vi "Transport Optimization Using Linear Programming.vi"() -> ()   [LabVIEW 2023]
doc: "Uses the Linear Programming Simplex Method VI to determine the number of units that company x transports to trader y."
panel:
  out "Error Status":bool
  in  "Tab Control":T1(tab)
  in  "Producers":cluster{"name":string, "produced units":dbl}[](array[cluster])=[{"name"="company A", "produced units"=213.0}, {"name"="company B", "produced units"=342.0}, {"name"="company C", "produced units"=543.0}, {"name"="company D", "produced units"=154.0}] {"produced units" format="%#.6g"}
  in  "Traders":cluster{"name":string, "needed units":dbl}[](array[cluster])=[{"name"="trader 1", "needed units"=564.0}, {"name"="trader 2", "needed units"=123.0}, {"name"="trader 3", "needed units"=234.0}, {"name"="trader 4", "needed units"=331.0}] {"needed units" format="%#.6g"}
  out "sum of produced units":dbl format="%#.6g"
  out "sum of needed units":dbl format="%#.6g"
  in  "Transport Costs (currency)":dbl[][](array[numeric])=[[213.0, 301.0, 453.0, 743.0], [99.0, 612.0, 209.0, 543.0], [123.0, 109.0, 453.0, 435.0], [129.0, 234.0, 432.0, 876.0]] min=0.0 format="%#.6g"
  out "Producers names":string[](array[string])
  out "Traders names":string[](array[string])
  out "minimal cost":dbl
  out "What delivers producer to trader #?":dbl[](graph)
  in  "Producer selector":u16(ring) items=["company A", "company B", "company C", "company D"]
  in  "Trader selector":u16(ring) items=["trader 1", "trader 2", "trader 3", "trader 4"]
  out "What gets trader from company #?":dbl[](graph)
  out "production":dbl
  out "delivery":dbl
  out "solution":dbl[][](array[numeric]) format="%#.2g"
  in  "Stop":bool
  # "Overview: Uses the Linear Programming Simplex Method VI to determine the number of units that company x transports to trader y with the firm M.\nRequirements: LabVIEW Full Development System\nInstructions: \n1. Specify the number of units in the Production and Consumption tab. Also, define the cost of transportation from each producer to each trader in the Transport Cost tab.\n2. Run the VI and verify the solution of this problem in the Solution tab. Use the Producer selector and Trader selector rings to analyze company and trader costs and minimum possible cost.\n3. Click Stop to stop the VI."
  # "Trader 1"
  # "Costs"
  # "P1->T1"
  # "Producer 1"
  # "P1->T2"
  # "Trader 2"
  # "Producer 2"
  # "P2->T1"
  # "P2->T2"
  # "Transporter"
  # "produced units"
  # "needed units"
  # "Constraint - every unit produced is consumed."
  # "The Transportation Problem is a linear programming problem where the lowest cost of transportation between Producer and Trader is obtained, taking into account the maximum throughput. The formulation is:\n\nMinimize: Sum ( c11.x11 + c12.x12 + .. + cmn.xmn).\nSubject to:\nx11 + x12 + ... + x1n <= b1;\n......\nxm1 + xm2 + ... + xmn <= bm;\nx11 + x12 + ... + xm1 >= a1;\n.......\nxm1 + xm2 + ... + xmn >= an;\nwhere:\nm: number of producers.\nn: number of traders."
  # "Traders"
  # "0"
  # "1"
  # "2"
  # "3"
  # "0"
  # "Producers"
  # "1"
  # "2"
  # "3"
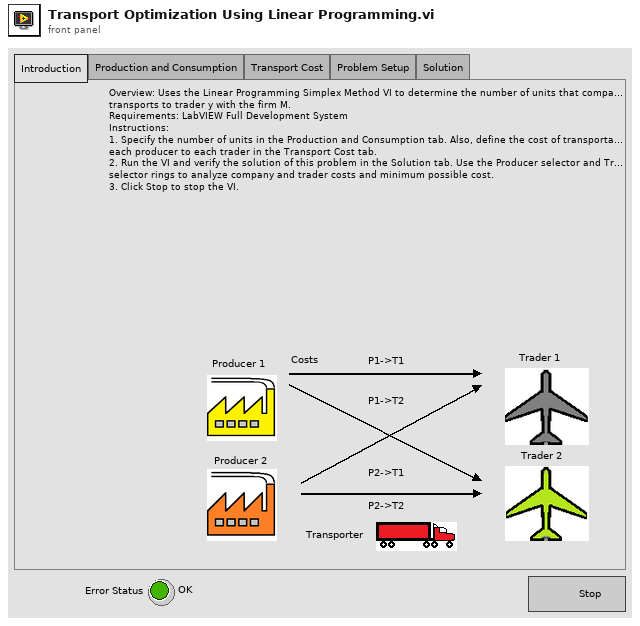
[diagram p1: front panel]
types:
  T1 = enum32{"Introduction", "Production and Consumption", "Transport Cost", "Problem Setup", "Solution"}
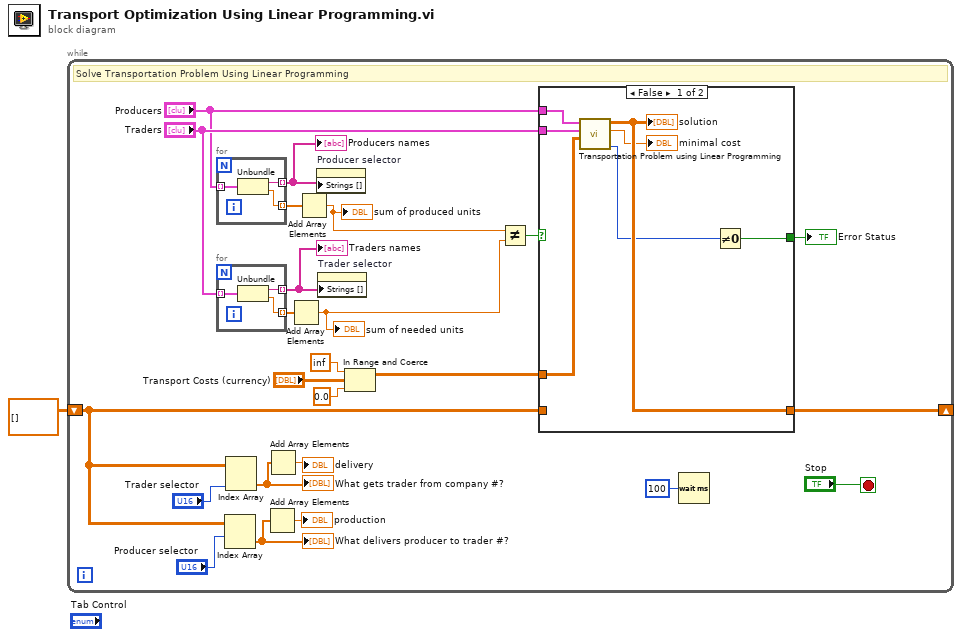
[diagram p0: block diagram]
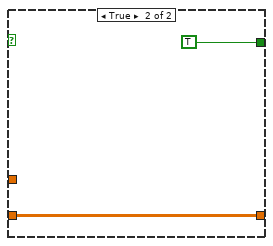
[diagram p2: hidden frame]
diagram:
  n1 = while {
    shift-left: dbl[][] [] ("Solution") -> [w5]
    shift-right: [w25] -> _
    stop <- "Stop" stop-if-true
    # "Solve Transportation Problem Using Linear Programming"
    n2 = for {
      tunnel: [w28] -> w8 mode=indexing
      tunnel: "Producers" -> [w27] mode=indexing
      tunnel: [w26] -> w10 mode=indexing
      n3 = Unbundle(w27) -> ("name"=w28:string, "produced units"=w26:dbl)
    }
    "Producers names" <- w8
    n4 = for {
      tunnel: [w40] -> w23 mode=indexing
      tunnel: "Traders" -> [w39] mode=indexing
      tunnel: [w38] -> w16 mode=indexing
      n5 = Unbundle(w39) -> ("name"=w40:string, "needed units"=w38:dbl)
    }
    "Traders names" <- w23
    n6 = Index Array(array=w5, index (row)="Producer selector") -> (element=w20:dbl[])  [unwired: 1 in]
    "What delivers producer to trader #?" <- w20
    n7 = Index Array(array=w5, index (col)="Trader selector") -> (element=w17:dbl[])  [unwired: 1 in]
    "What gets trader from company #?" <- w17
    n8 = Add Array Elements(numeric array=w20) -> (sum=→"production":dbl)
    n9 = Add Array Elements(numeric array=w17) -> (sum=→"delivery":dbl)
    n10 = Add Array Elements(numeric array=w16) -> (sum=w15:dbl)
    "sum of needed units" <- w15
    n11 = Add Array Elements(numeric array=w10) -> (sum=w14:dbl)
    "sum of produced units" <- w14
    n12 = property on="Producer selector" class="Ring (strict)"("Strings []"=w8) -> ()  [unwired: 2 in, 2 out]
    n13 = property on="Trader selector" class="Ring (strict)"("Strings []"=w23) -> ()  [unwired: 2 in, 2 out]
    n14 = In Range and Coerce(upper limit=inf, x="Transport Costs (currency)", lower limit=0.0) -> (coerced(x)=w11:dbl[][])  [unwired: 1 out]
    n15 = Not Equal?(x=w14, y=w15) -> (x != y?=w4:bool)
    n16 = case shown="False" w4 {
      tunnel: "Traders" -> [w35 _]
      tunnel: [w34 w37] -> w25
      tunnel: "Producers" -> [w32 _]
      tunnel: w5 -> [_ w37]
      tunnel: w11 -> [w31 _]
      tunnel: [w30 TRUE ("Error")] -> w6
      frame False {
        n17 = call "Transportation Problem using Linear Programming.vi"("Transport Costs"=w31, "Traders"=w35, "Producers"=w32) -> ("error"=w29:i32, "minimal cost"=→"minimal cost":dbl, "Solution"=w34:dbl[][])  [unwired: 6 in]
        "solution" <- w34
        n18 = Not Equal To 0?(x=w29) -> (x != 0?=w30:bool)
      }
      frame True {
      }
    }
    "Error Status" <- w6
    n19 = Wait (ms)(milliseconds to wait=u32 100) -> ()  [unwired: 1 out]
  }
